vi "LSX Get Hdi Speed Index.vi"(0 "lLSID":i32, 1 "plA":i32, 5 "plX":i32, 7 "plY":i32, 9 "plZ":i32, 11 "error in (no error)":errorcluster) -> (3 "plA out":i32, 4 "function return":i32, 6 "plX out":i32, 8 "plY out":i32, 10 "plZ out":i32, 15 "error out":errorcluster)   [LabVIEW 2016, in "Tango_DLL.lvlib"]
doc: "TANGOAPI int TANGOCALL LSX_GetHdiSpeedIndex (int lLSID, int *plX, int *plY, int *plZ, int *plA);"
uses:
  Tango_DLL.lvlib
  2017/Microscope Control/Device Library/Stages/Marzhauser/SCAN IM 120 x 80/Tango DLL VIs/Tango_DLL.dll
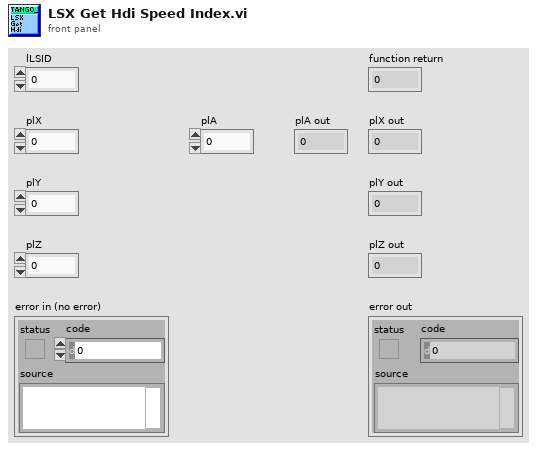
[diagram p1: front panel]
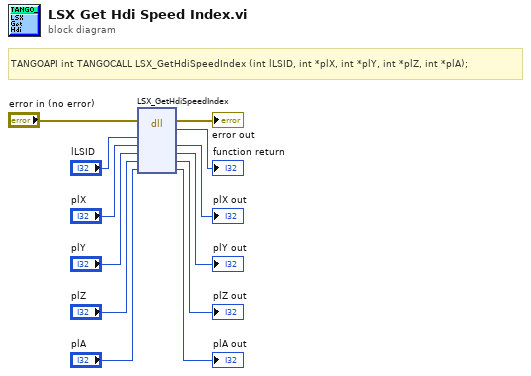
[diagram p0: block diagram]
diagram:
  # "TANGOAPI int TANGOCALL LSX_GetHdiSpeedIndex (int lLSID, int *plX, int *plY, int *plZ, int *plA);"
  n1 = dll-call lib="C:/Users/4PiSMS/Documents/Microscope Control/2017/Microscope Control/Device Library/Stages/Marzhauser/SCAN IM 120 x 80/Tango DLL VIs/Tango_DLL.*" fn="LSX_GetHdiSpeedIndex"(error in="error in (no error)", "lLSID"="lLSID", "plX"="plX", "plY"="plY", "plZ"="plZ", "plA"="plA") -> (error out=→"error out":errorcluster, →"function return":i32, "plX"=→"plX out":i32, "plY"=→"plY out":i32, "plZ"=→"plZ out":i32, "plA"=→"plA out":i32)  [unwired: 3 in, 1 out]
